vi "AlarmLoop.vi"(8 "Error In":errorcluster, 9 "ABLE Configuration":T1, 10 "ABLE Data Structures":T7, 11 "Action Queues":T8) -> (0 "Error Out":errorcluster)   [LabVIEW 2012]
doc: "This VI controls the alarms displayed on the Alarms screen of the graphical user interface."
uses:
  ActionQueues.ctl
  UIActionQueueElement.ctl
  UIAction.ctl
  HardwareActionQueueElement.ctl
  HardwareAction.ctl
  ExperimentActionQueueElement.ctl
  ExperimentAction.ctl
  AlarmQueueElement.ctl
  AlarmAction.ctl
  ABLEDataStructures.ctl
  HardwareDisplayData.ctl
  BPM.ctl
  ExperimentHardwareData.ctl
  ExperimentData.ctl
  AlarmData.ctl
  AlarmDatum.ctl
  ABLEConfiguration.ctl
  DisplayConfiguration.ctl
  FolderConfiguration.ctl
  AlarmsConfiguration.ctl
  Keithley6485Configuration.ctl
  Keithley6482Configuration.ctl
  AlarmSetups.ctl
  AlarmSetup.ctl
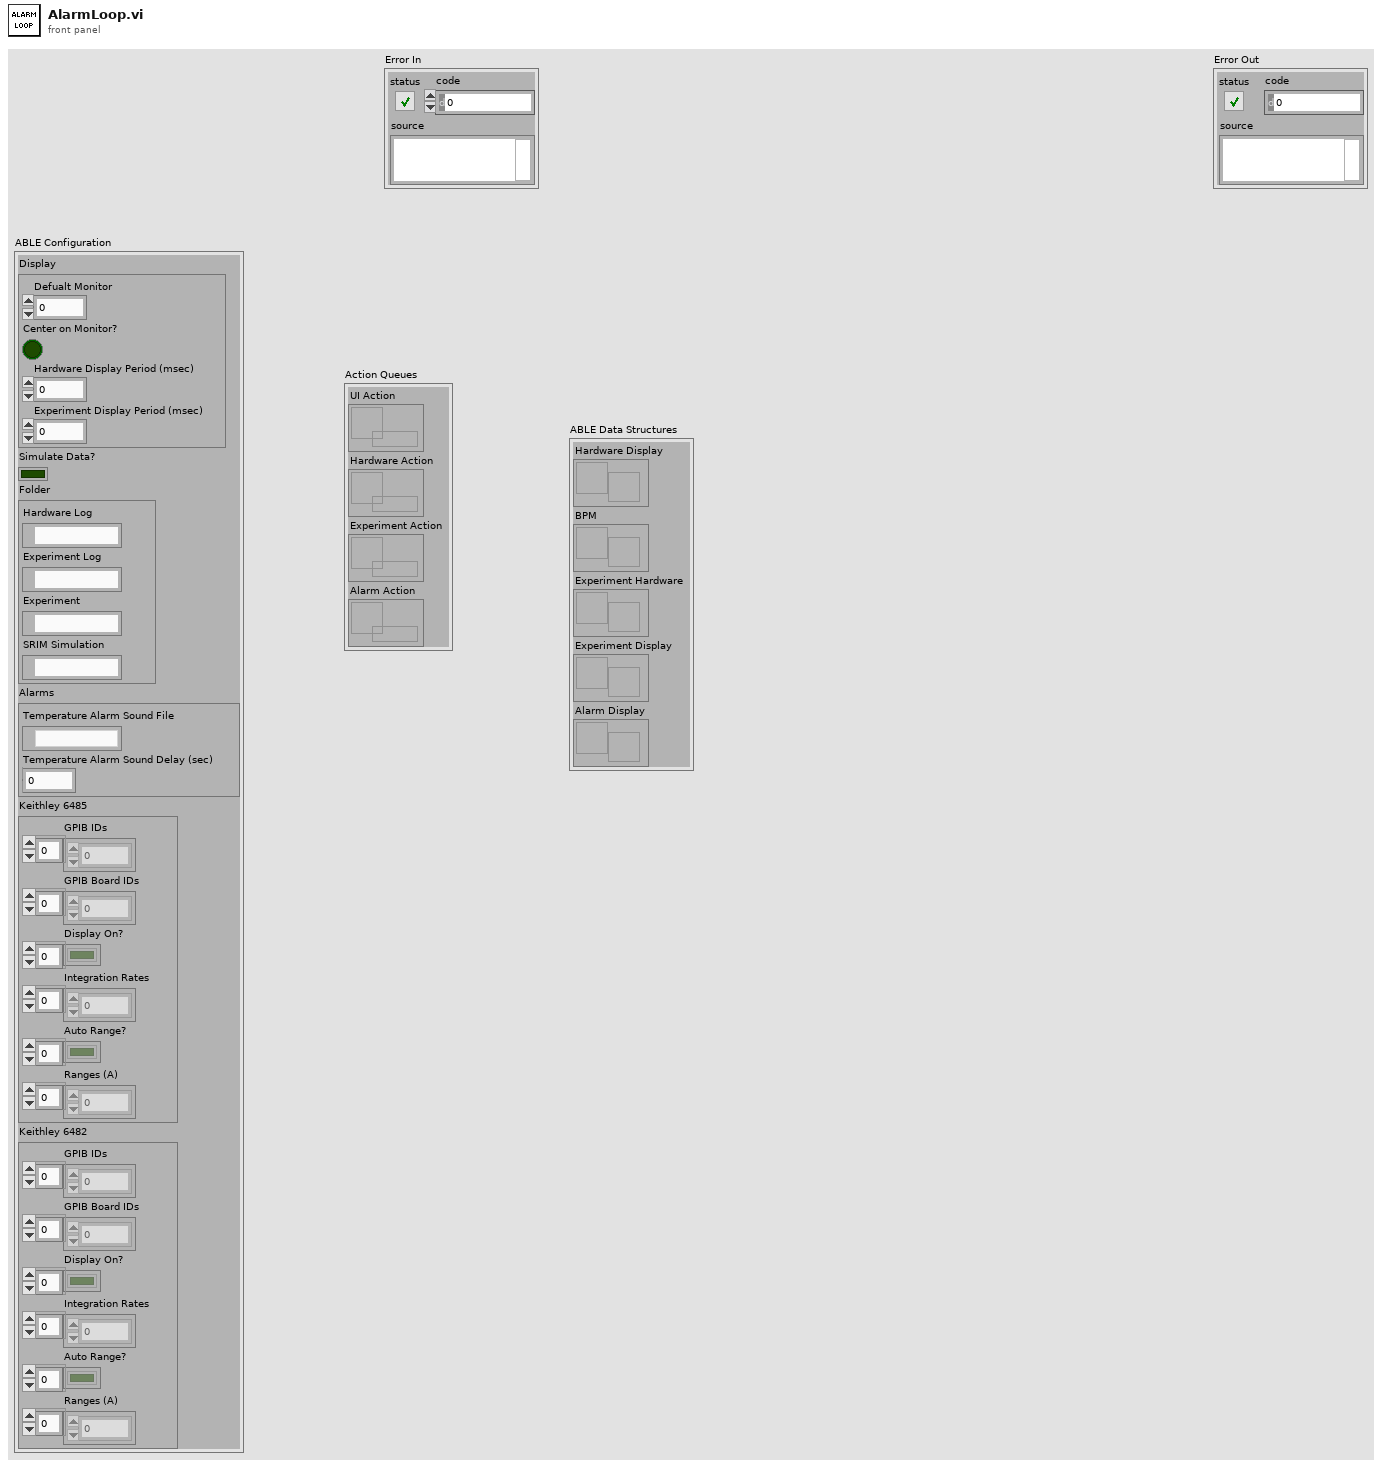
[diagram p1: front panel]
types:
  T1 = typedef "ABLEConfiguration.ctl" = cluster{"Display":T2, "Simulate Data?":bool, "Folder":T3, "Alarms":T4, "Keithley 6485":T5, "Keithley 6482":T6}
  T2 = typedef "DisplayConfiguration.ctl" = cluster{"Defualt Monitor":u16, "Center on Monitor?":bool, "Hardware Display Period (msec)":u32, "Experiment Display Period (msec)":u32}
  T3 = typedef "FolderConfiguration.ctl" = cluster{"Hardware Log":path, "Experiment Log":path, "Experiment":path, "SRIM Simulation":path}
  T4 = typedef "AlarmsConfiguration.ctl" = cluster{"Temperature Alarm Sound File":path, "Temperature Alarm Sound Delay (sec)":dbl}
  T5 = typedef "Keithley6485Configuration.ctl" = cluster{"GPIB IDs":u8[], "GPIB Board IDs":u8[], "Display On?":bool[], "Integration Rates":dbl[], "Auto Range?":bool[], "Ranges (A)":dbl[]}
  T6 = typedef "Keithley6482Configuration.ctl" = cluster{"GPIB IDs":u8[], "GPIB Board IDs":u8[], "Display On?":bool[], "Integration Rates":dbl[], "Auto Range?":bool[], "Ranges (A)":dbl[]}
  T7 = typedef "ABLEDataStructures.ctl" = cluster{"Hardware Display":refnum<notifier>, "BPM":refnum<notifier>, "Experiment Hardware":refnum<notifier>, "Experiment Display":refnum<notifier>, "Alarm Display":refnum<notifier>}
  T8 = typedef "ActionQueues.ctl" = cluster{"UI Action":refnum<queue>, "Hardware Action":refnum<queue>, "Experiment Action":refnum<queue>, "Alarm Action":refnum<queue>}
  T9 = typedef "AlarmSetups.ctl" = cluster{"Temperature":T10[]}
  T10 = typedef "AlarmSetup.ctl" = cluster{"ENABLED":bool, "High Limit":dbl, "Low Limit":dbl}
  T11 = typedef "AlarmQueueElement.ctl" = cluster{"Action":T12, "Data":variant}
  T12 = typedef "AlarmAction.ctl" = enum16{"Initialize", "Load", "Check", "Shutdown"}
  T13 = typedef "AlarmData.ctl" = cluster{"Temperature":T14[]}
  T14 = typedef "AlarmDatum.ctl" = cluster{"Actual":dbl, "Activated?":bool}
  T15 = typedef "HardwareDisplayData.ctl" = cluster{"Temperatures (C)":dbl[], "Terminal Voltage (MeV)":dbl, "Currents (A)":dbl[]}
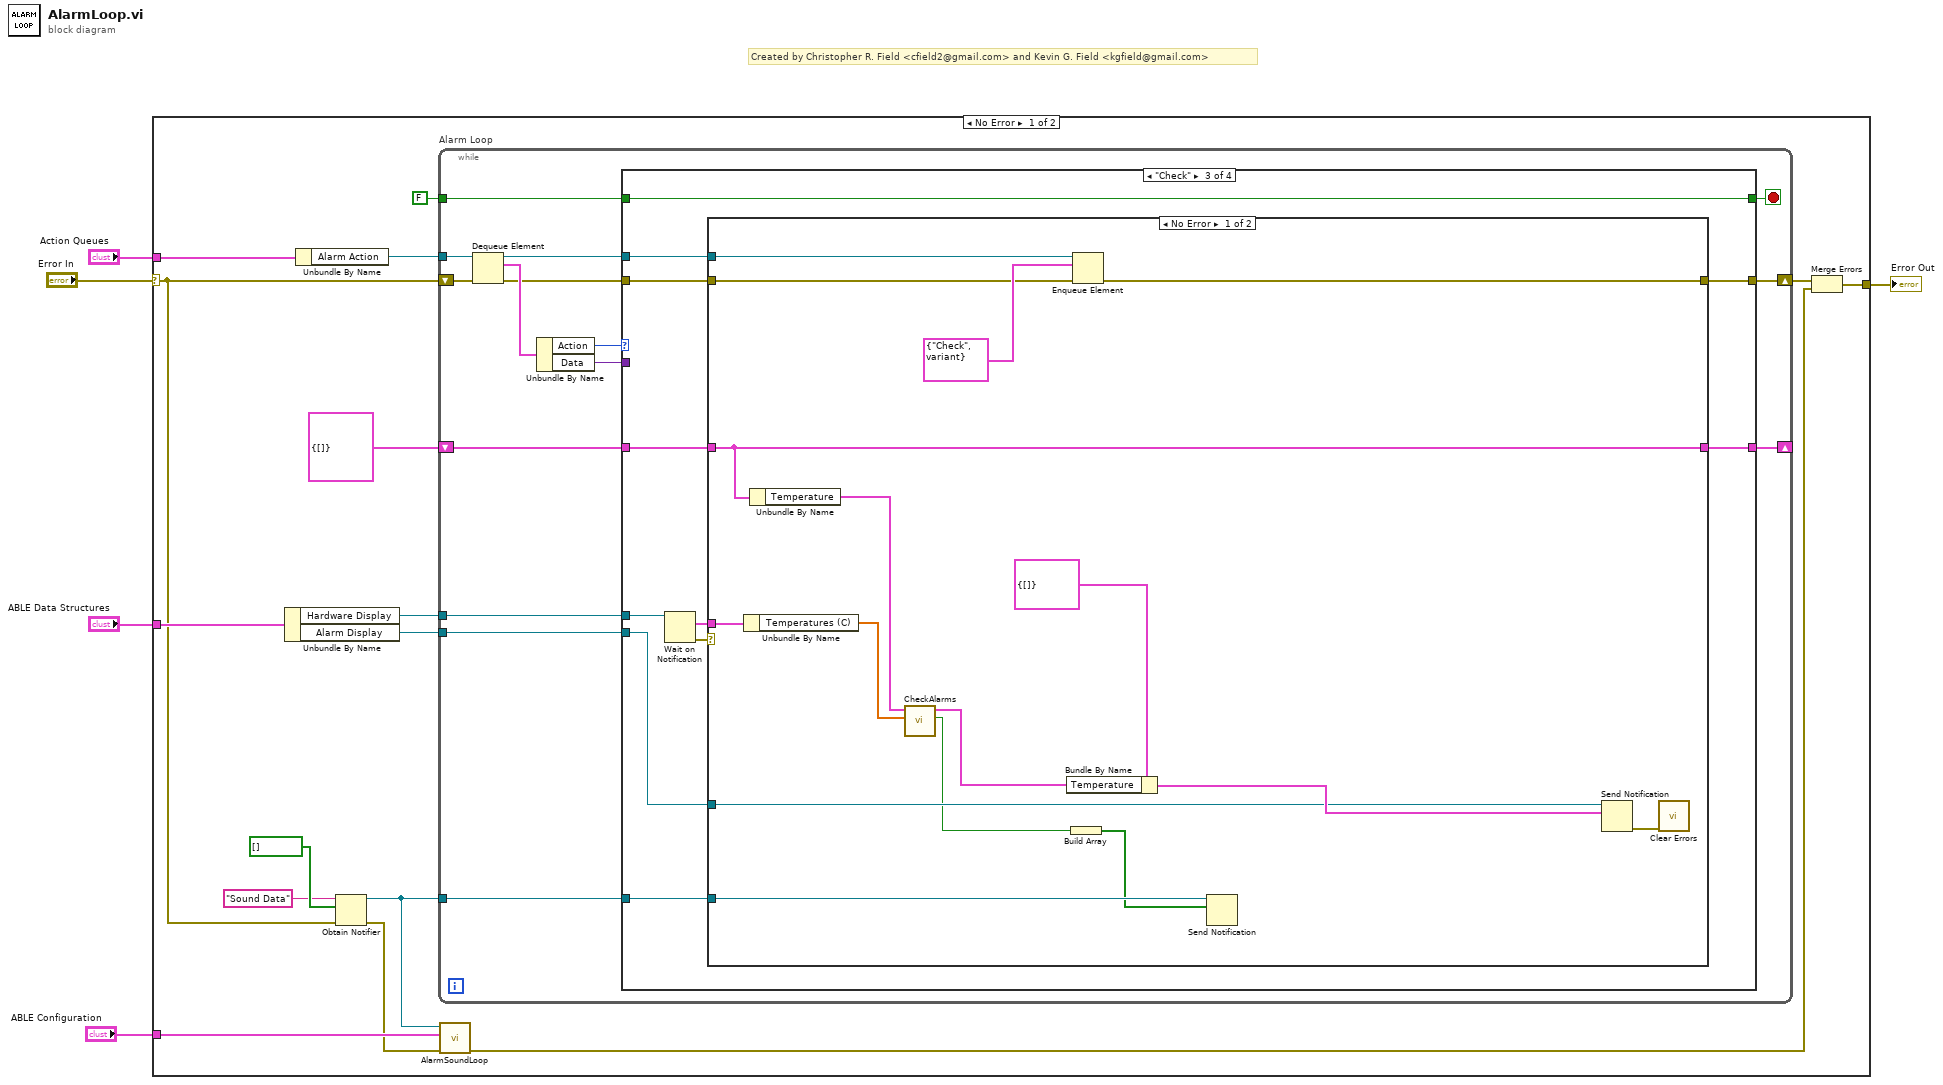
[diagram p0: block diagram]
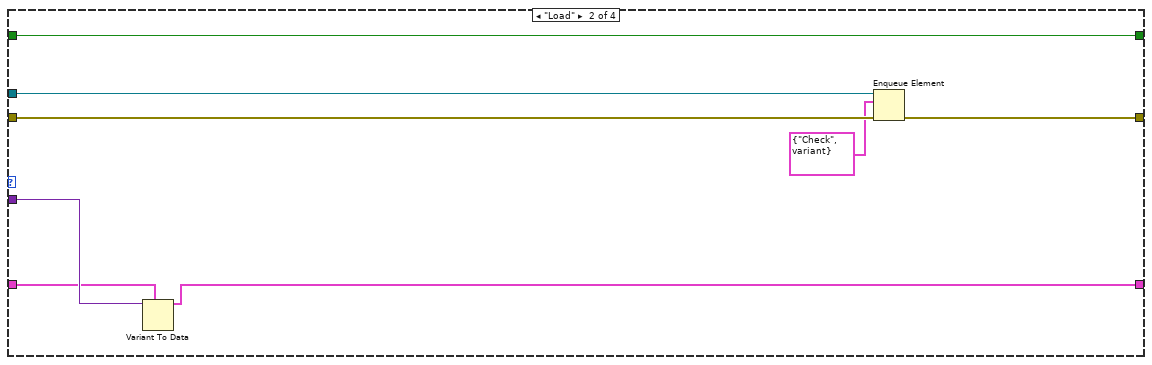
[diagram p3: hidden frame]
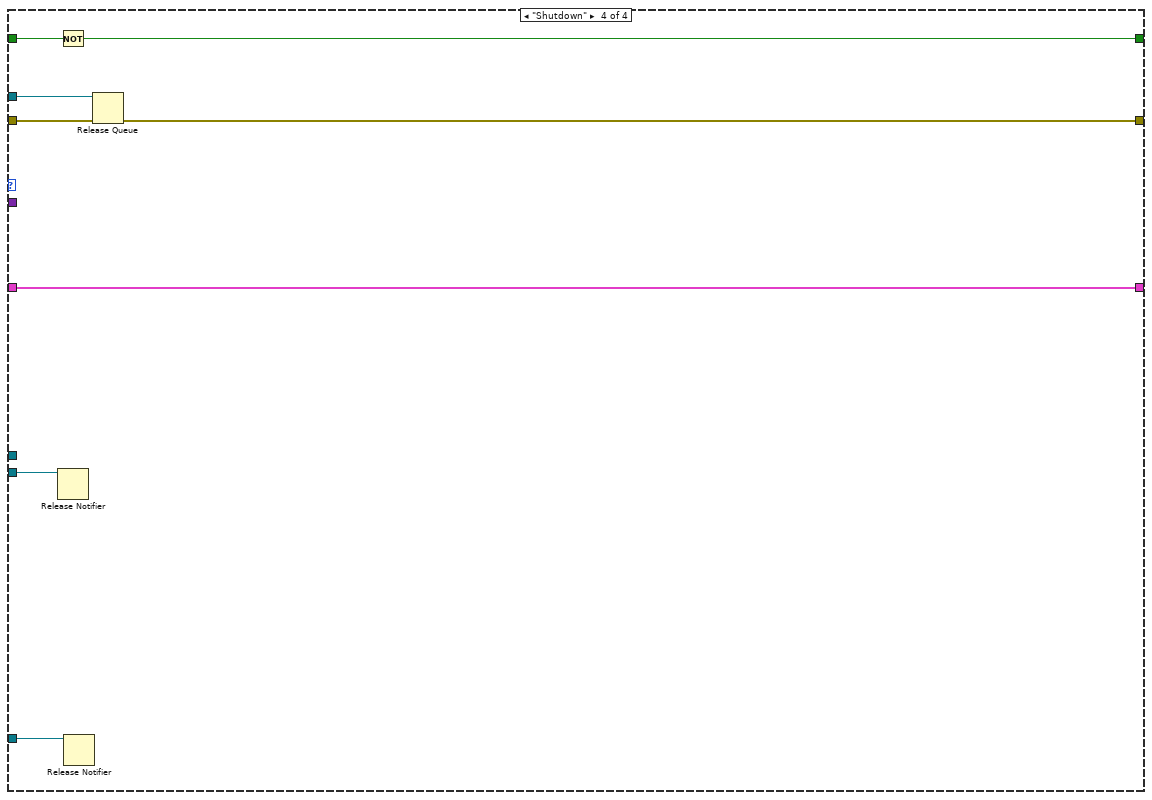
[diagram p5: hidden frame]
diagram:
  # "Created by Christopher R. Field <cfield2@gmail.com> and Kevin G. Field <kgfield@gmail.com>"
  n1 = case shown="No Error" "Error In" {
    selector: "Error In" -> [w7 w85]
    tunnel: "Action Queues" -> [w21 _]
    tunnel: [w12 w85] -> w3
    tunnel: "ABLE Data Structures" -> [w18 _]
    tunnel: "ABLE Configuration" -> [w14 _]
    frame No Error {
      n2 = Unbundle By Name(w18) -> ("Hardware Display"=w17:refnum<notifier>, "Alarm Display"=w16:refnum<notifier>)
      n3 = Unbundle By Name(w21) -> ("Alarm Action"=w20:refnum<queue>)
      n4 = Obtain Notifier(name (unnamed)="Sound Data", notification data type=bool[] [], error in (no error)=w7) -> (notifier out=w6:refnum<notifier>, error out=w8:errorcluster)  [unwired: 1 in, 1 out]
      n5 = while "Alarm Loop" {
        shift-right: [w29] -> w13
        shift-left: w7 -> [w35]
        tunnel: w20 -> [w36]
        tunnel: FALSE -> [w28]
        tunnel: w17 -> [w26]
        shift-right: [w24] -> _
        shift-left: T9 {"Temperature"=[]} ("Alarm Setups") -> [w25]
        tunnel: w16 -> [w23]
        tunnel: w6 -> [w22]
        stop <- w27 stop-if-true
        n6 = Dequeue Element(queue=w36, error in (no error)=w35) -> (queue out=w31:refnum<queue>, element=w34:T11, error out=w32:errorcluster)  [unwired: 1 in, 1 out]
        n7 = Unbundle By Name(w34) -> ("Action"=w33:T12, "Data"=w30:variant)
        n8 = case shown="\"Check\"" w33 {
          tunnel: w32 -> [w37 w45 w50 w80]
          tunnel: w31 -> [_ w46 w52 w81]
          tunnel: w30 -> [_ w42 _ _]
          tunnel: [w37 w44 w51 w79] -> w29
          tunnel: w28 -> [w39 w47 w58 w84]
          tunnel: [w39 w47 w58 w83] -> w27
          tunnel: w26 -> [_ _ w57 _]
          tunnel: w25 -> [w38 w41 w55 w82]
          tunnel: [w38 w40 w49 w82] -> w24
          tunnel: w23 -> [_ _ w54 w77]
          tunnel: w22 -> [_ _ w48 w78]
          frame "Initialize", Default {
          }
          frame "Load" {
            n9 = Variant To Data(type=w41, Variant=w42) -> (data=w40:T9)  [unwired: 1 in, 1 out]
            n10 = Enqueue Element(queue=w46, element=T11 {"Action"=enum."Check", "Data"=variant}, error in (no error)=w45) -> (error out=w44:errorcluster)  [unwired: 1 in, 2 out]
          }
          frame "Check" {
            n11 = Wait on Notification(notifier=w57) -> (notification=w56:T15, error out=w53:errorcluster)  [unwired: 3 in, 2 out]
            n12 = case shown="No Error" w53 {
              tunnel: w56 -> [w74 _]
              tunnel: w55 -> [w63 w75]
              tunnel: w54 -> [w68 _]
              tunnel: w52 -> [w67 _]
              tunnel: [w66 w76] -> w51
              tunnel: w50 -> [w64 w76]
              tunnel: [w63 w75] -> w49
              tunnel: w48 -> [w60 _]
              frame No Error {
                n13 = Unbundle By Name(w74) -> ("Temperatures (C)"=w72:dbl[])
                n14 = Unbundle By Name(w63) -> ("Temperature"=w73:T10[])
                n15 = call "CheckAlarms.vi"("Values"=w72, "Alarm Setups"=w73) -> ("Alarm Tripped?"=w61:bool, "Alarm Data"=w70:T14[])  [unwired: 8 in]
                n16 = Bundle By Name(cluster=T13 {"Temperature"=[]} ("Alarm Data"), "Temperature"=w70) -> (w69:T13)
                n17 = Build Array(w61) -> (w59:bool[])
                n18 = Enqueue Element(queue=w67, element=T11 {"Action"=enum."Check", "Data"=variant}, error in (no error)=w64) -> (error out=w66:errorcluster)  [unwired: 1 in, 2 out]
                n19 = Send Notification(notification=w59, notifier=w60) -> ()  [unwired: 1 in, 2 out]
                n20 = Send Notification(notification=w69, notifier=w68) -> (error out=w62:errorcluster)  [unwired: 1 in, 1 out]
                n21 = call <vilib>:"Clear Errors.vi"("error in (no error)"=w62) -> ()  [unwired: 6 in, 1 out]
              }
              frame Error {
              }
            }
          }
          frame "Shutdown" {
            n22 = Not(x=w84) -> (.not. x?=w83:bool)
            n23 = Release Notifier(notifier=w77) -> ()  [unwired: 2 in, 3 out]
            n24 = Release Notifier(notifier=w78) -> ()  [unwired: 2 in, 3 out]
            n25 = Release Queue(queue=w81, error in (no error)=w80) -> (error out=w79:errorcluster)  [unwired: 1 in, 2 out]
          }
        }
      }
      n26 = call "AlarmSoundLoop.vi"("Error In"=w8, "ABLE Configuration"=w14, "Sound Data"=w6) -> ("Error Out"=w11:errorcluster)  [unwired: 8 in]
      n27 = Merge Errors(w13, w11) -> (w12:errorcluster)
    }
    frame Error {
    }
  }
  "Error Out" <- w3
